vi "Format countdown.vi"(10 "Elapsed (sec)":i64, 11 "Countdown total (min)":i64) -> (3 "Formatted countdown":string)   [LabVIEW 2015]
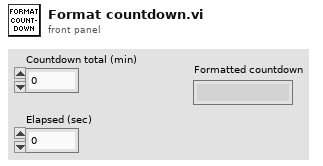
[diagram p1: front panel]
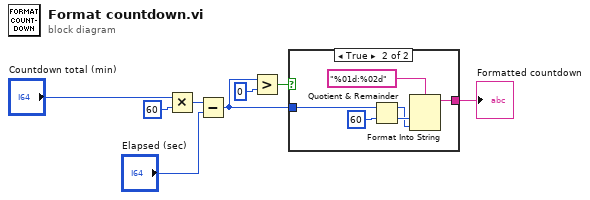
[diagram p0: block diagram]
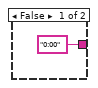
[diagram p2: hidden frame]
diagram:
  n1 = Multiply(x="Countdown total (min)", y=i64 60) -> (x*y=w6:i64)
  n2 = Subtract(x=w6, y="Elapsed (sec)") -> (x-y=w1:i64)
  n3 = Greater?(x=w1, y=i64 0) -> (0:w3:bool)
  n4 = case shown="True" w3 {
    tunnel: ["0:00" w10] -> w2
    tunnel: w1 -> [_ w15]
    frame False {
    }
    frame True {
      n5 = Quotient & Remainder(x=w15, y=i64 60) -> (x-y*floor(x/y)=w11:i64, floor(x/y)=w12:i64)
      n6 = Format Into String(format string="%01d:%02d", w12, w11) -> (resulting string=w10:string)  [unwired: 2 in, 1 out]
    }
  }
  "Formatted countdown" <- w2
